vi "Maximum Single Tick Time.vi"() -> (0 "Maximum Single Tick (s)":dbl)   [LabVIEW 2015]
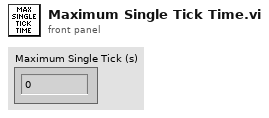
[diagram p1: front panel]
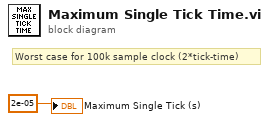
[diagram p0: block diagram]
diagram:
  # "Worst case for 100k sample clock (2*tick-time)"
  "Maximum Single Tick (s)" <- 2e-05 ("low time")
